vi "Run main.vi"() -> ()   [LabVIEW 2016]
uses:
  Program Files (x86)/National Instruments/LabVIEW 2016/examples/robotics/EPOS2 CANOpen Driver/Low Level VIs/Typedefs/CAN Refnum.ctl
  Program Files (x86)/National Instruments/LabVIEW 2016/examples/robotics/EPOS2 CANOpen Driver/Low Level VIs/Typedefs/CAN Session Pointer.ctl
  Program Files (x86)/National Instruments/LabVIEW 2016/examples/robotics/EPOS2 CANOpen Driver/Low Level VIs/Typedefs/CAN Communication References.ctl
  Program Files (x86)/National Instruments/LabVIEW 2016/examples/robotics/EPOS2 CANOpen Driver/Low Level VIs/Typedefs/kill process notifier array.ctl
  Program Files (x86)/National Instruments/LabVIEW 2016/examples/robotics/EPOS2 CANOpen Driver/Low Level VIs/Typedefs/Write Queue.ctl
  Program Files (x86)/National Instruments/LabVIEW 2016/examples/robotics/EPOS2 CANOpen Driver/Low Level VIs/Typedefs/FPGA CAN Frame Cluster.ctl
  RT/BMS Voltage status 2.ctl
  Tests/BMS Status.ctl
  RT/Pedals Status.ctl
  RT/Clustered SDO.ctl
  RT/Statusword.ctl
  Tests/Dashboard Control.ctl
  RT/Battery Status.ctl
  Tests/Log File Cluster.ctl
  <vilib>/Platform/TimedLoop/XDataNode/timing_clust.ctl
  <vilib>/Platform/TimedLoop/XDataNode/nitl_modes.ctl
  <vilib>/Platform/TimedLoop/XDataNode/wakeup.ctl
  <vilib>/Platform/TimedLoop/XDataNode/XDataNode.xnode
  <vilib>/Platform/TimedLoop/XDataNode/XDNodeRunTimeDep.lvlib
  <vilib>/NI_Real-Time Target Support.lvlib
  <vilib>/RTwatchdog.llb/Watchdog expiration actions.ctl
panel:
  out "Error Notifier":refnum<notifier>
  out "LED Period":i64
  out "LED Color":i16
  out "Last Pedals Update":u32
  in  "Tab Control":T1(tab)
  in  "Don't irritate me":bool=TRUE
  in  "Simulate BMS LV":bool=TRUE
  in  "Simulate Dashboard":bool=TRUE
  in  "Simulate Pedals":bool=TRUE
  in  "Simulate Motors":bool=TRUE
  in  "Simulation Interval":u32=20
  in  "Simulate BMS":bool=TRUE
  in  "\"Pedals\" Status":T2 {"Acceleration pedal" scale=0.0..100.0 scale format="%#_6f%%"; "Break pedal" scale=0.0..100.0 scale format="%#_6f%%"}
  out "Left Motor Status":T3
  out "Target Torque Left":i16(knob) scale=-1000.0..1000.0
  out "Left Motor Statusword":T4
  out "Right Motor Status":T3
  out "Right Motor Statusword":T4
  out "Target Torque Right":i16(knob) scale=1000.0..-1000.0
  out "BMS Status":T5
  out "Battery Status":T6
  out "BMS Low Voltage Status":T7 {"Temp. 0" scale=0.0..80.0; "Temp. 1" scale=0.0..80.0}
  in  "Ready to drive":bool
  in  "Simulate Pumps":bool
  in  "Pumps power":dbl(slide) scale=0.0..100.0 scale format="%#_g%%"
  in  "Dashboard Control":T8={"Tractive System"=TRUE, "RTD"=TRUE, "AMS error"=TRUE, "IMD error"=TRUE, "Low Voltage"=0.0, "High Voltage"=0.0} {"High Voltage" scale=0.0..10.0; "Low Voltage" scale=0.0..10.0}
  in  "Error Listbox":i32(listbox)
  out "Update motors notifier":i32
  out "Update Motors Notifier":refnum<notifier>
  out "Emergency Turn Off Notifier":refnum<notifier>
  out "Pedals status":i32
  out "Update motors":i32
  out "Pool status":i32
  out "Error Queue":refnum<queue>
  out "Shutdown Notifier":refnum<notifier>
  out "Log File Cluster":T9
  out "CAN Session":T11
  out "CANOpen Session":refnum<k20>
  out "Left motor Clustered SDO":T12
  out "Right motor Clustered SDO":T12
  out "State Ring":u16(ring) items=["Init VI", "Init Event Handlers", "Booting sequence", "Operational", "Emergency shutting down", "Shuting down", "Closing VI"]
  in  "Emergency Shutdown Button":bool
  in  "Shutdown Button":bool
  in  "Stop":bool
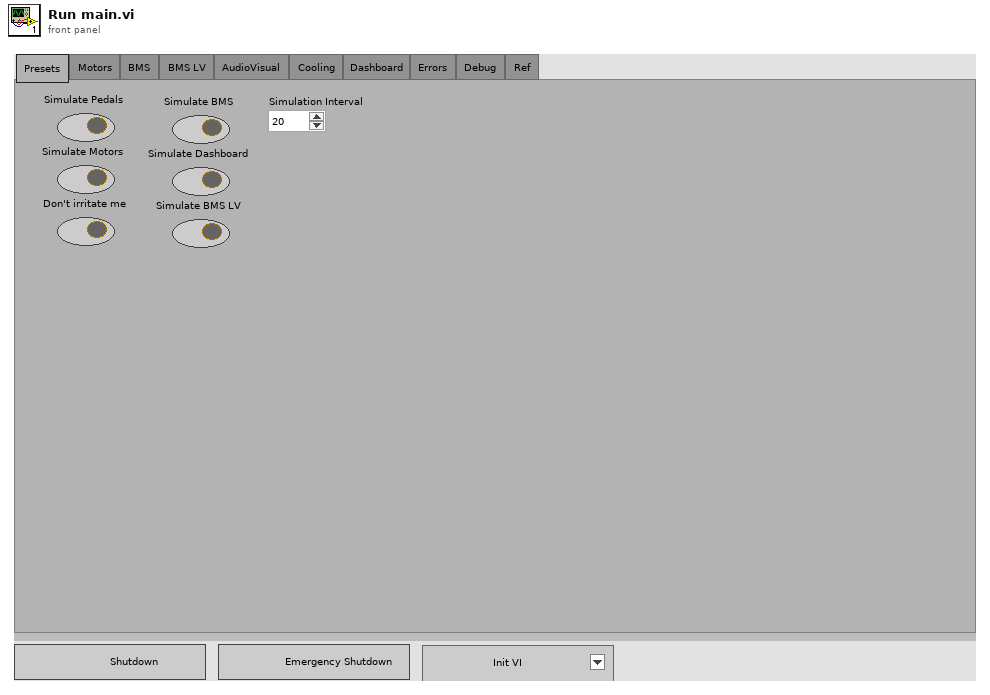
[diagram p1: front panel]
types:
  T1 = enum32{"Presets ", "Motors ", "BMS ", "BMS LV ", "AudioVisual ", "Cooling ", "Dashboard", "Errors ", "Debug ", "Ref "}
  T2 = typedef "Pedals Status.ctl" = cluster{"Acceleration pedal":dbl, "Break pedal":dbl, "Sterring wheel":dbl[unit]}
  T3 = cluster{"Statusword":u16, "Warnings":u16, "Error code":u16, "Error register":u8, "Controller temperature":u8, "Motor temperature":u8, "Troque actual value":i16, "Velocity actual value":i32, "Electric power":u32, "DC current":u32, "Phase A current":u16, "Phase B current":u16, "Electrical Angle":u16}
  T4 = typedef "Statusword.ctl" = cluster{"Ready to switch on":bool, "Switched on":bool, "Operation enabled":bool, "Fault":bool, "Voltage enabled":bool, "Quick stop":bool, "Switch on disabled":bool, "Warning":bool, "Remote":bool, "Target reached":bool, "Internal limit active":bool, "Operation mode specific":bool, "Manufacturer specific":bool}
  T5 = typedef "BMS Status.ctl" = cluster{"INIT":bool, "READY":bool, "WAIT_FOR_ACTIVE":bool, "ACTIVE":bool, "ERROR":bool}
  T6 = typedef "Battery Status.ctl" = cluster{"Hall sensor":i32, "Percent of charge":i16}
  T7 = typedef "BMS Voltage status 2.ctl" = cluster{"Cells Voltage":dbl[], "Temp. 1":u8, "Temp. 0":u8}
  T8 = typedef "Dashboard Control.ctl" = cluster{"Tractive System":bool, "RTD":bool, "AMS error":bool, "IMD error":bool, "Low Voltage":dbl, "High Voltage":dbl}
  T9 = typedef "Log File Cluster.ctl" = cluster{"Log file":refnum<k34>, "semaphore":T10}
  T10 = typedef "Semaphore RefNum" = refnum<k1>
  T11 = typedef "CAN Refnum.ctl" = refnum<k1>
  T12 = typedef "Clustered SDO.ctl" = cluster{"SDO object out":refnum<k20>, "semaphore":T10}
  T13 = typedef "Watchdog expiration actions.ctl" = cluster{"reset":bool, "occurrence":bool, "trigger protocol":enum16{"active high", "active low", "open collector"}, "trigger line":enum16{"none", "line 0", "line 1", "line 2", "line 3", "line 4", "line 5", "line 6", "line 7", "SMB line 0"}, "disable watchdog on VI exit":bool}
  T14 = typedef "XDNodeRunTimeDep.lvlib/timing_clust.ctl" = cluster{"Expected End [f-1]":u64, "Actual End [f-1]":u64, "Finished Late? [f-1]":bool, "Expected End [i-1]":u64, "Actual End [i-1]":u64, "Finished Late? [i-1]":bool, "Expected Start [i]":u64, "Actual Start [i]":u64, "Expected Start [f]":u64, "Actual Start [f]":u64, "Source Name":string, "Structure Name":string, "Period":i64, "Deadline":i64, "Offset":i64, "Start":i64, "Priority":i32, "Timeout":i32, "Mode":T15, "Wakeup Reason":T16, "Error":errorcluster, "Source Type":string, "Secondary Source Type":string, "Global End Time":u64, "Global Start Time":u64, "Frame Duration":u64, "Iteration Duration":u64, "Assigned CPU":i32, "I/O Scan Engine Mode":u32}
  T15 = typedef "XDNodeRunTimeDep.lvlib/nitl_modes.ctl" = enum32{"No Change", "Process missed periods, maintain original phase", "Discard missed periods, maintain original phase", "Process missed periods, ignore original phase", "Discard missed periods, ignore original phase"}
  T16 = typedef "XDNodeRunTimeDep.lvlib/wakeup.ctl" = enum32{"Normal", "Aborted", "Asynchronous wakeup", "Timing source error", "Timed loop error", "Timeout"}
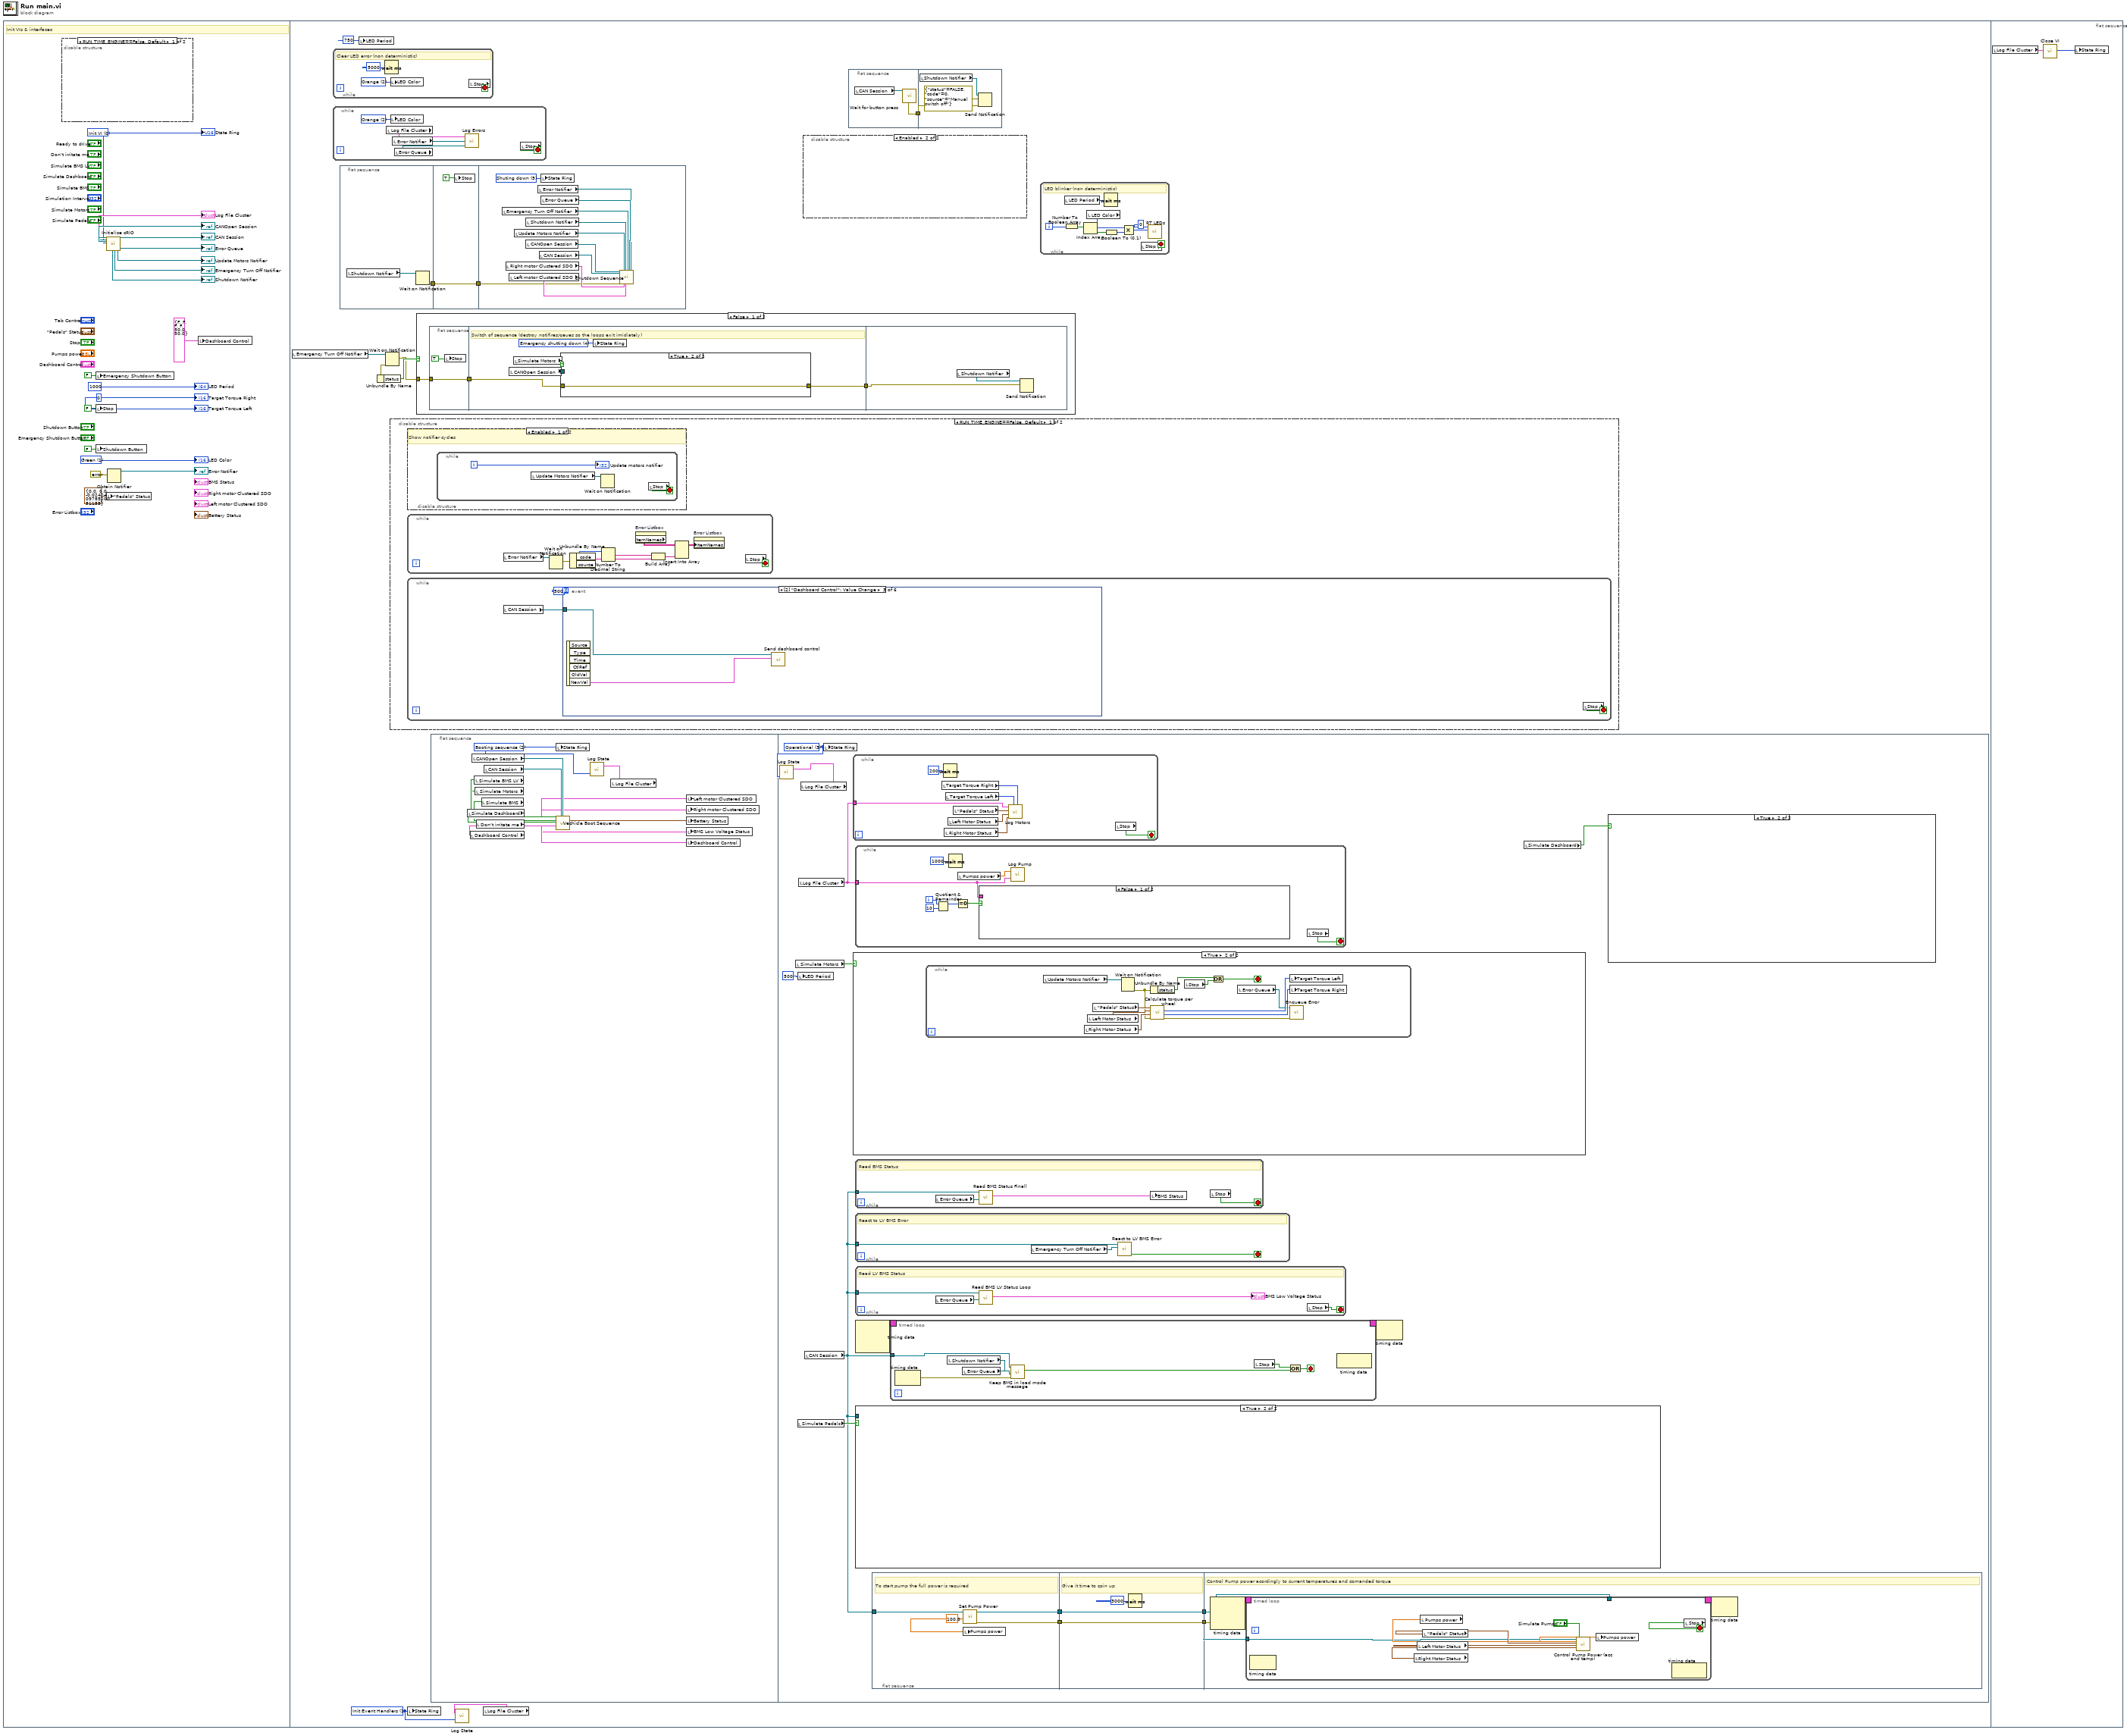
[diagram p0: block diagram]
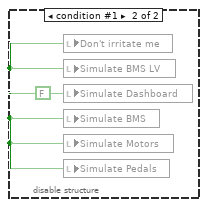
[diagram p2: hidden frame]
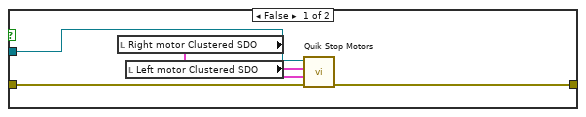
[diagram p3: hidden frame]
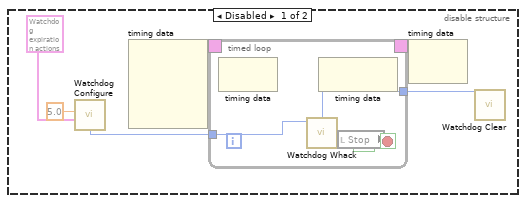
[diagram p5: hidden frame]
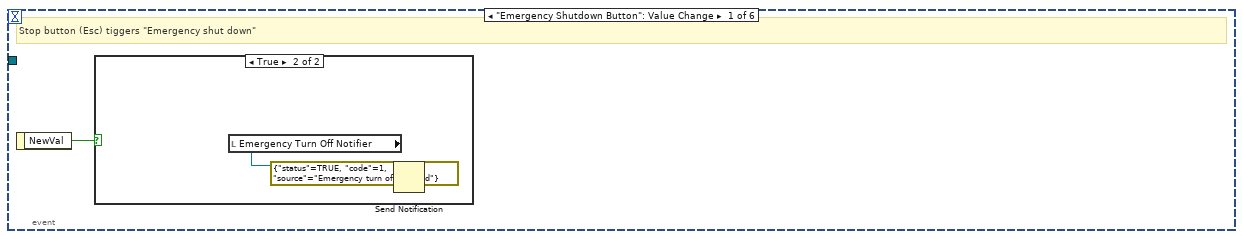
[diagram p7: hidden frame]
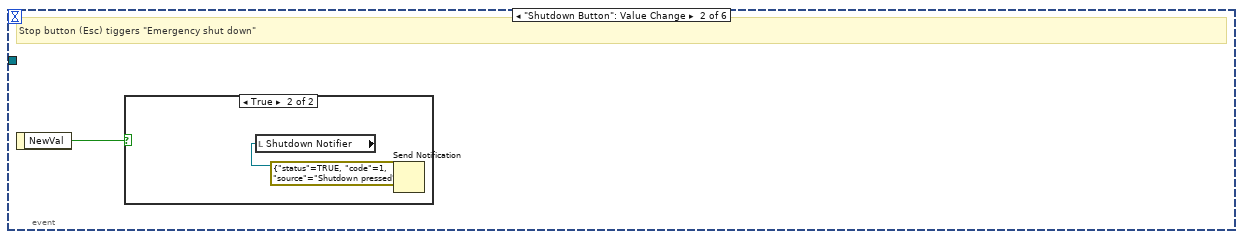
[diagram p9: hidden frame]
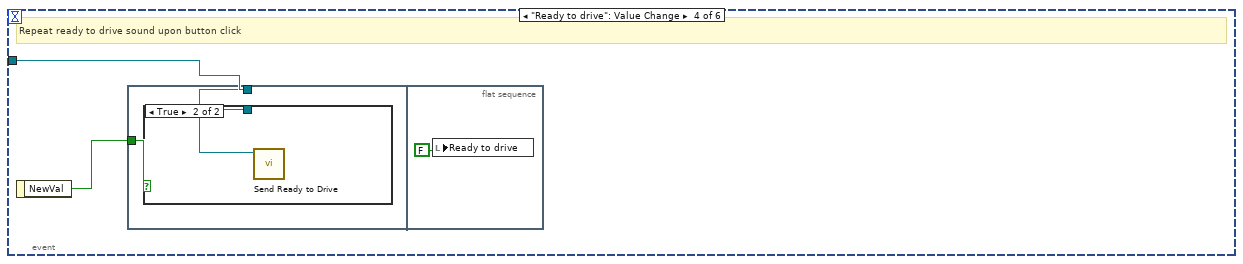
[diagram p11: hidden frame]
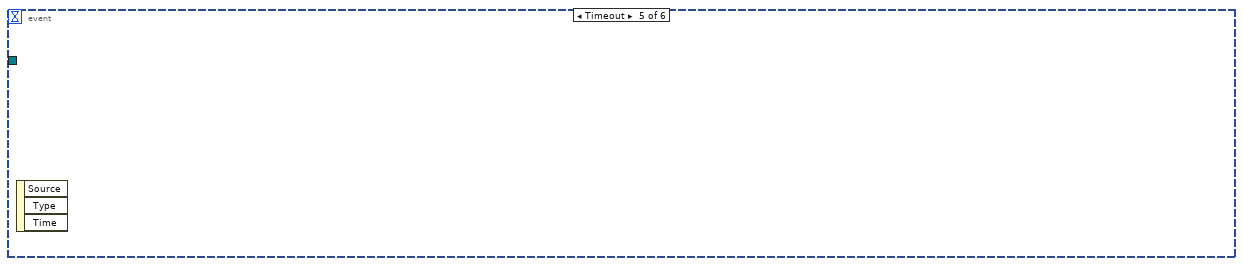
[diagram p13: hidden frame]
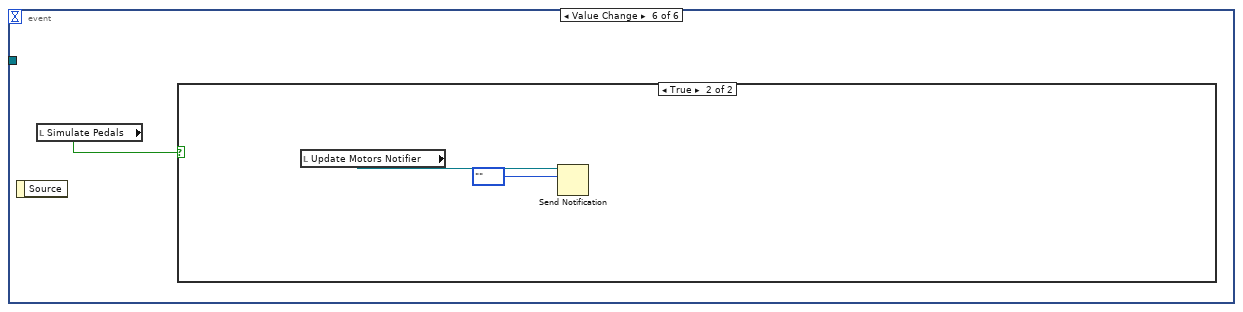
[diagram p14: hidden frame]
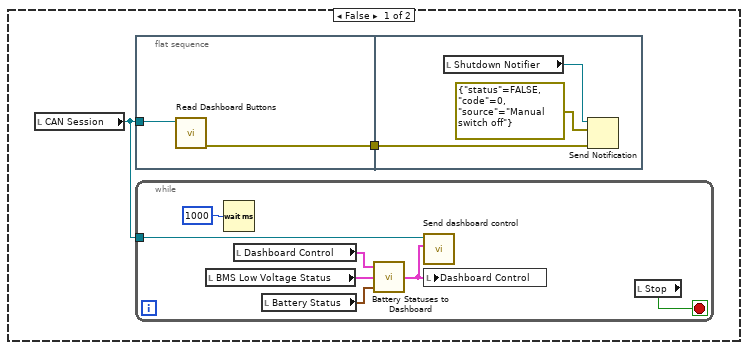
[diagram p17: hidden frame]
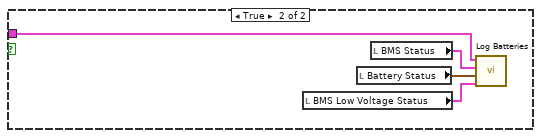
[diagram p18: hidden frame]
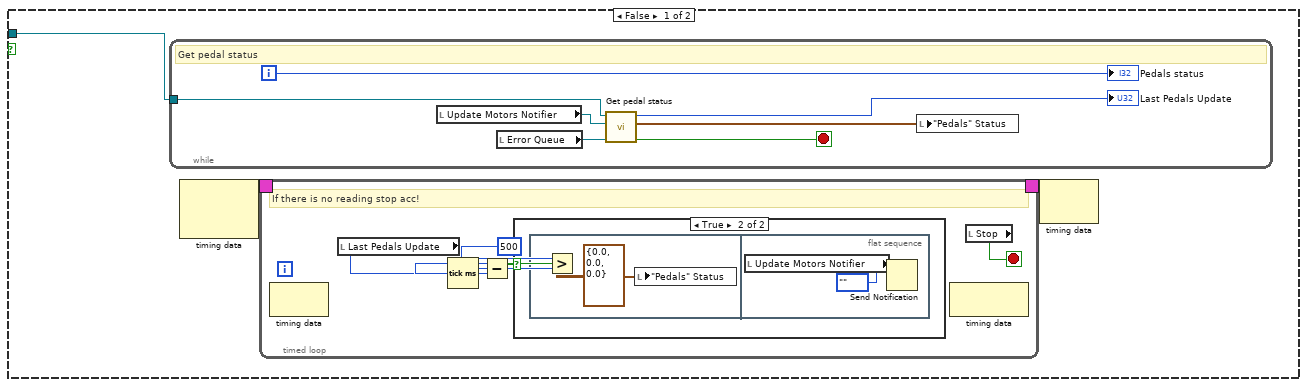
[diagram p19: hidden frame]
diagram:
  n1 = flat-sequence {
    frame #0 {
      w2 = u16 0 items=["Init VI", "Init Event Handlers", "Booting sequence", "Operational", "Emergency shutting down", "Shuting down", "Closing VI"] ("State Ring")
      w10 = u16 1 items=["Green"=1, "Orange"=2]
      w12 = i16 0 ("Target Torque")
      # "Init VIs & interfaces"
      n2 = disable-structure shown="RUN_TIME_ENGINE==False, Default" {
        frame condition #0 (active) {
        }
        frame condition #1 {
          w19 = FALSE ("Don't irritate me")
          n3 = local write "Don't irritate me"(w19) -> ()
          n4 = local write "Simulate BMS LV"(w19) -> ()
          n5 = local write "Simulate Dashboard"(w19) -> ()
          n6 = local write "Simulate BMS"(w19) -> ()
          n7 = local write "Simulate Motors"(w19) -> ()
          n8 = local write "Simulate Pedals"(w19) -> ()
        }
      }
      n9 = local write "Emergency Shutdown Button"(FALSE ("Emergency Shutdown Button")) -> ()
      n10 = local write "Stop"(FALSE ("Stop")) -> ()
      n11 = local write "Shutdown Button"(FALSE ("Shutdown Button")) -> ()
      n12 = call "Initialise cRIO.vi"("State Ring"=w2) -> ("Shutdown Notifier"=→"Shutdown Notifier":refnum<notifier>, "Emergency Turn Off Notifier"=→"Emergency Turn Off Notifier":refnum<notifier>, "Update Motors Notifier"=→"Update Motors Notifier":refnum<notifier>, "Log File Cluster"=→"Log File Cluster":T9, "CANOpen Session"=→"CANOpen Session":refnum<k20>, "CAN Session"=→"CAN Session":T11, "Error Queue"=→"Error Queue":refnum<queue>)  [unwired: 19 in, 1 out]
      n13 = local write "\"Pedals\" Status"(T2 {"Acceleration pedal"=0.0, "Break pedal"=0.0, "Sterring wheel"=-0.024240978520051155} ("\"Pedals\" Status")) -> ()
      n14 = Obtain Notifier(notification data type=errorcluster {"status"=FALSE, "code"=0, "source"=""} ("error constant")) -> (notifier out=→"Error Notifier":refnum<notifier>)  [unwired: 3 in, 2 out]
      n15 = local write "Dashboard Control"(T8 {"Tractive System"=FALSE, "RTD"=FALSE, "AMS error"=FALSE, "IMD error"=FALSE, "Low Voltage"=50.0, "High Voltage"=50.0} ("Dashboard Control")) -> ()
      "Target Torque Left" <- w12
      "Target Torque Right" <- w12
      "LED Color" <- w10
      "LED Period" <- i64 1000 ("LED Period")
      "State Ring" <- w2
    }
    frame #1 {
      w27 = u16 1 items=["Init VI", "Init Event Handlers", "Booting sequence", "Operational", "Emergency shutting down", "Shuting down", "Closing VI"] ("State Ring")
      n16 = local read "Emergency Turn Off Notifier"() -> (w23:refnum<notifier>)
      n17 = while {
        stop <- w76 stop-if-true
        w77 = u16 2 items=["Green"=1, "Orange"=2]
        # "Clear LED error (non deterministic)"
        n18 = Wait (ms)(milliseconds to wait=u32 5000) -> ()  [unwired: 1 out]
        n19 = local write "LED Color"(w77) -> ()
        n20 = local read "Stop"() -> (w76:bool)
      }
      n21 = while {
        stop <- w82 stop-if-true
        w80 = u16 2 items=["Green"=1, "Orange"=2]
        n22 = local read "Log File Cluster"() -> (w79:T9)
        n23 = local write "LED Color"(w80) -> ()
        n24 = local read "Error Notifier"() -> (w78:refnum<notifier>)
        n25 = local read "Error Queue"() -> (w81:refnum<queue>)
        n26 = call "Log Errors.vi"("Error Queue"=w81, "Error Notifier"=w78, "Log File Cluster"=w79) -> ()  [unwired: 1 in]
        n27 = local read "Stop"() -> (w82:bool)
      }
      n28 = flat-sequence {
        tunnel: [w115] -> w25
        tunnel: w25 -> [w118]
        tunnel: [w118] -> w24
        tunnel: w24 -> [w123]
        frame #0 {
          n29 = local read "Shutdown Notifier"() -> (w116:refnum<notifier>)
          n30 = Wait on Notification(notifier=w116) -> (error out=w115:errorcluster)  [unwired: 3 in, 3 out]
        }
        frame #1 {
          n31 = local write "Stop"(TRUE ("Stop")) -> ()
        }
        frame #2 {
          w120 = u16 5 items=["Init VI", "Init Event Handlers", "Booting sequence", "Operational", "Emergency shutting down", "Shuting down", "Closing VI"] ("State Ring")
          n32 = local read "Emergency Turn Off Notifier"() -> (w121:refnum<notifier>)
          n33 = local read "Right motor Clustered SDO"() -> (w124:T12)
          n34 = local read "Left motor Clustered SDO"() -> (w125:T12)
          n35 = local read "Update Motors Notifier"() -> (w127:refnum<notifier>)
          n36 = local read "Shutdown Notifier"() -> (w126:refnum<notifier>)
          n37 = local read "CANOpen Session"() -> (w129:refnum<k20>)
          n38 = local read "Error Notifier"() -> (w119:refnum<notifier>)
          n39 = local read "CAN Session"() -> (w128:T11)
          n40 = local write "State Ring"(w120) -> ()
          n41 = local read "Error Queue"() -> (w122:refnum<queue>)
          n42 = call "Shutdown Sequence.vi"("CANOpen Session"=w129, "CAN Session"=w128, "error in (no error)"=w123, "Update Motors Notifier"=w127, "Right motor Clustered SDO"=w124, "Shutdown Notifier"=w126, "Left motor Clustered SDO"=w125, "Emergency Turn Off Notifier"=w121, "Error Queue"=w122, "Error Notifier"=w119) -> ()  [unwired: 17 in, 1 out]
        }
      }
      n43 = local write "LED Period"(i64 750 ("LED Period")) -> ()
      n44 = Wait on Notification(notifier=w23) -> (notification=w20:errorcluster, error out=w22:errorcluster)  [unwired: 3 in, 2 out]
      n45 = Unbundle By Name(w22) -> ("status"=w21:bool)
      n46 = disable-structure shown="RUN_TIME_ENGINE==False, Default" {
        frame condition #0 (active) {
          n47 = disable-structure shown="Enabled" {
            frame Enabled {
              # "Show notifier cycles"
              n48 = while {
                i -> [w92]
                stop <- w93 stop-if-true
                n49 = local read "Update Motors Notifier"() -> (w94:refnum<notifier>)
                n50 = Wait on Notification(notifier=w94) -> ()  [unwired: 3 in, 4 out]
                n51 = local read "Stop"() -> (w93:bool)
                "Update motors notifier" <- w92
              }
            }
            frame Disabled {
            }
          }
          n52 = while {
            stop <- w83 stop-if-true
            n53 = local read "Error Notifier"() -> (w91:refnum<notifier>)
            n54 = Wait on Notification(notifier=w91) -> (notification=w90:errorcluster)  [unwired: 3 in, 3 out]
            n55 = Unbundle By Name(w90) -> ("code"=w87:i32, "source"=w89:string)
            n56 = Number To Decimal String(number=w87) -> (decimal integer string=w88:string)  [unwired: 1 in]
            n57 = property on="Error Listbox" class="MCListbox (strict)"() -> ("ItemNames"=w85:string[][])  [unwired: 2 in, 2 out]
            n58 = Build Array(w88, w89) -> (w86:string[])
            n59 = Insert Into Array(array=w85, new element=w86) -> (w84:string[][])  [unwired: 2 in]
            n60 = property on="Error Listbox" class="MCListbox (strict)"("ItemNames"=w84) -> ()  [unwired: 2 in, 2 out]
            n61 = local read "Stop"() -> (w83:bool)
          }
          n62 = while {
            stop <- w96 stop-if-true
            n63 = local read "CAN Session"() -> (w97:T11)
            n64 = event shown="[2] \"Dashboard Control\": Value Change" {
              selector: _ -> [_ _ _ _ _ _]
              dyn-events: _ -> [_ _ _ _ _ _]
              timeout: 500 -> [_ _ _ _ _ _]
              tunnel: w97 -> [_ _ w104 w106 _ _]
              event "Emergency Shutdown Button": Value Change {
                # "Stop button (Esc) tiggers \"Emergency shut down\""
                n65 = event-data() -> ("NewVal"=w98:bool)  [unwired: 1 in]
                n66 = case shown="True" w98 {
                  frame False {
                  }
                  frame True {
                    n67 = local read "Emergency Turn Off Notifier"() -> (w100:refnum<notifier>)
                    n68 = Send Notification(notification=errorcluster {"status"=TRUE, "code"=1, "source"="Emergency turn off pressed"}, notifier=w100) -> ()  [unwired: 1 in, 2 out]
                  }
                }
              }
              event "Shutdown Button": Value Change {
                # "Stop button (Esc) tiggers \"Emergency shut down\""
                n69 = event-data() -> ("NewVal"=w101:bool)  [unwired: 1 in]
                n70 = case shown="True" w101 {
                  frame False {
                  }
                  frame True {
                    n71 = local read "Shutdown Notifier"() -> (w103:refnum<notifier>)
                    n72 = Send Notification(notification=errorcluster {"status"=TRUE, "code"=1, "source"="Shutdown pressed"}, notifier=w103) -> ()  [unwired: 1 in, 2 out]
                  }
                }
              }
              event Value Change {
                n73 = event-data() -> ("NewVal"=w105:T8)  [unwired: 1 in, 5 out]
                n74 = call "Send dashboard control.vi"("Dashboard Control"=w105, "CAN Session In"=w104) -> ()  [unwired: 8 in, 2 out]
              }
              event "Ready to drive": Value Change {
                # "Repeat ready to drive sound upon button click"
                n75 = event-data() -> ("NewVal"=w107:bool)  [unwired: 1 in]
                n76 = flat-sequence {
                  tunnel: w107 -> [w109]
                  tunnel: w106 -> [w108]
                  frame #0 {
                    n77 = case shown="True" w109 {
                      tunnel: w108 -> [_ w110]
                      frame False {
                      }
                      frame True {
                        n78 = call "Send Ready to Drive.vi"("CAN Session In"=w110) -> ()  [unwired: 9 in, 2 out]
                      }
                    }
                  }
                  frame #1 {
                    n79 = local write "Ready to drive"(FALSE ("Ready to drive")) -> ()
                  }
                }
              }
              event Timeout {
                n80 = event-data() -> ()  [unwired: 1 in, 3 out]
              }
              event Value Change {
                n81 = event-data() -> ()  [unwired: 1 in, 1 out]
                n82 = local read "Simulate Pedals"() -> (w112:bool)
                n83 = case shown="True" w112 {
                  frame False {
                  }
                  frame True {
                    n84 = local read "Update Motors Notifier"() -> (w113:refnum<notifier>)
                    n85 = Send Notification(notification=enum16{""}."", notifier=w113) -> ()  [unwired: 1 in, 2 out]
                  }
                }
              }
            }
            n86 = local read "Stop"() -> (w96:bool)
          }
        }
        frame condition #1 {
        }
      }
      n87 = local write "State Ring"(w27) -> ()
      n88 = case shown="False" w21 {
        tunnel: w20 -> [w30 _]
        frame False {
          n89 = flat-sequence {
            tunnel: [w33] -> w32
            tunnel: w30 -> [w33]
            tunnel: w32 -> [w35]
            tunnel: [w37] -> w31
            tunnel: w31 -> [w46]
            frame #0 {
              n90 = local write "Stop"(TRUE ("Stop")) -> ()
            }
            frame #1 {
              w36 = u16 4 items=["Init VI", "Init Event Handlers", "Booting sequence", "Operational", "Emergency shutting down", "Shuting down", "Closing VI"] ("State Ring")
              # "Switch of sequence (destroy notifires/qeues so the loops exit imidiately)"
              n91 = local read "CANOpen Session"() -> (w38:refnum<k20>)
              n92 = local read "Simulate Motors"() -> (w39:bool)
              n93 = case shown="True" w39 {
                tunnel: w38 -> [w44 _]
                tunnel: [w41 w45] -> w37
                tunnel: w35 -> [w40 w45]
                frame False {
                  n94 = local read "Right motor Clustered SDO"() -> (w42:T12)
                  n95 = local read "Left motor Clustered SDO"() -> (w43:T12)
                  n96 = call "Quik Stop Motors.vi"("error in (no error)"=w40, "Left motor Clustered SDO"=w43, "Right motor Clustered SDO"=w42, "CANOpen session"=w44) -> ("error out"=w41:errorcluster)  [unwired: 5 in, 2 out]
                }
                frame True {
                }
              }
              n97 = local write "State Ring"(w36) -> ()
            }
            frame #2 {
              n98 = local read "Shutdown Notifier"() -> (w47:refnum<notifier>)
              n99 = Send Notification(notification=w46, notifier=w47) -> ()  [unwired: 1 in, 2 out]
            }
          }
        }
        frame True {
        }
      }
      n100 = flat-sequence {
        frame #0 {
          w131 = u16 2 items=["Init VI", "Init Event Handlers", "Booting sequence", "Operational", "Emergency shutting down", "Shuting down", "Closing VI"] ("State Ring")
          n101 = local read "Simulate Dashboard"() -> (w141:bool)
          n102 = local read "Dashboard Control"() -> (w133:T8)
          n103 = local read "CANOpen Session"() -> (w138:refnum<k20>)
          n104 = local read "Simulate BMS LV"() -> (w144:bool)
          n105 = local read "Simulate Motors"() -> (w142:bool)
          n106 = local read "Don't irritate me"() -> (w140:bool)
          n107 = local read "Simulate BMS"() -> (w143:bool)
          n108 = local read "CAN Session"() -> (w139:T11)
          n109 = local write "State Ring"(w131) -> ()
          n110 = call "Vechicle Boot Sequence.vi"("Simulate BMS LV"=w144, "Simulate Motors"=w142, "Simulate BMS"=w143, "Simulate Dashboard"=w141, "Don't irritate me"=w140, "Dashboard Control in"=w133, "CAN Session"=w139, "CANOpen Session"=w138) -> ("Left motor Clustered SDO"=w136:T12, "Right motor Clustered SDO"=w137:T12, "Battery Status"=w135:T6, "BMS Low Voltage Status"=w132:T7, "Dashboard Control out"=w134:T8)  [unwired: 14 in, 1 out]
          n111 = local read "Log File Cluster"() -> (w130:T9)
          n112 = call "Log State.vi"("State Ring"=w131, "Log File Cluster"=w130) -> ()  [unwired: 1 in]
          n113 = local write "Left motor Clustered SDO"(w136) -> ()
          n114 = local write "Right motor Clustered SDO"(w137) -> ()
          n115 = local write "Battery Status"(w135) -> ()
          n116 = local write "BMS Low Voltage Status"(w132) -> ()
          n117 = local write "Dashboard Control"(w134) -> ()
        }
        frame #1 {
          w146 = u16 3 items=["Init VI", "Init Event Handlers", "Booting sequence", "Operational", "Emergency shutting down", "Shuting down", "Closing VI"] ("State Ring")
          n118 = local read "Simulate Motors"() -> (w152:bool)
          n119 = local read "Simulate Pedals"() -> (w151:bool)
          n120 = local write "LED Period"(i64 500 ("LED Period")) -> ()
          n121 = local read "Log File Cluster"() -> (w148:T9)
          n122 = local read "Log File Cluster"() -> (w147:T9)
          n123 = call "Log State.vi"("State Ring"=w146, "Log File Cluster"=w147) -> ()  [unwired: 1 in]
          n124 = local read "CAN Session"() -> (w150:T11)
          n125 = local write "State Ring"(w146) -> ()
          n126 = while {
            tunnel: w148 -> [w185]
            stop <- w186 stop-if-true
            n127 = local read "Target Torque Right"() -> (w188:i16)
            n128 = Wait (ms)(milliseconds to wait=u32 200) -> ()  [unwired: 1 out]
            n129 = local read "Right Motor Status"() -> (w190:T3)
            n130 = local read "Target Torque Left"() -> (w189:i16)
            n131 = local read "Left Motor Status"() -> (w191:T3)
            n132 = local read "\"Pedals\" Status"() -> (w192:T2)
            n133 = call "Log Motors.vi"("Target Torque Right"=w188, "Target Torque Left"=w189, "Right Motor Status"=w190, "Left Motor Status"=w191, "\"Pedals\" Status"=w192, "Log File Cluster"=w185) -> ()  [unwired: 4 in]
            n134 = local read "Stop"() -> (w186:bool)
          }
          n135 = case shown="True" w152 {
            frame False {
              n136 = local read "Right motor Clustered SDO"() -> (w266:T12)
              n137 = local read "Left motor Clustered SDO"() -> (w267:T12)
              n138 = while {
                tunnel: w267 -> [w287]
                tunnel: w266 -> [w288]
                i -> [w290]
                stop <- w281 stop-if-true
                # "Update motors target values"
                n139 = local read "Update Motors Notifier"() -> (w289:refnum<notifier>)
                n140 = local read "Right Motor Status"() -> (w284:T3)
                n141 = local read "Left Motor Status"() -> (w285:T3)
                n142 = local read "\"Pedals\" Status"() -> (w286:T2)
                n143 = call "Update motors target values.vi"("Update Motors Notifier"=w289, "Right motor Clustered SDO"=w288, "Left motor Clustered SDO"=w287, "\"Pedals\" Status"=w286, "Left Motor Status"=w285, "Right Motor Status"=w284) -> ("Target Torque Left"=w283:i16, "Target Torque Right"=w282:i16, "Exit?"=w281:bool)  [unwired: 19 in]
                n144 = local write "Target Torque Left"(w283) -> ()
                n145 = local write "Target Torque Right"(w282) -> ()
                "Update motors" <- w290
              }
              n146 = node-c288() -> (w265:T14)  [unwired: 3 in]
              n147 = timed-loop {
                timing: w265 -> [_]
                timing-out: [_] -> w264
                tunnel: w267 -> [w275]
                tunnel: w266 -> [w274]
                i -> [w276]
                stop <- w268 stop-if-true
                # "Pool motor status"
                n148 = node-c288() -> ()  [unwired: 1 in, 2 out]
                n149 = local read "Update Motors Notifier"() -> (w273:refnum<notifier>)
                n150 = call "Pool motor status.vi"("Update Motors Notifier"=w273, "Right motor Clustered SDO"=w274, "Left motor Clustered SDO"=w275) -> ("Left Motor Status"=→"Left Motor Status":T3, "Left Motor Statusword"=→"Left Motor Statusword":T4, "Right Motor Status"=→"Right Motor Status":T3, "Right Motor Statusword"=→"Right Motor Statusword":T4, "Exit?"=w268:bool)  [unwired: 20 in]
                n151 = node-c288() -> ()  [unwired: 1 in, 1 out]
                "Pool status" <- w276
              }
              n152 = node-c288(w264) -> ()  [unwired: 1 out]
            }
            frame True {
              n153 = while {
                stop <- w298 stop-if-true
                n154 = local read "Update Motors Notifier"() -> (w300:refnum<notifier>)
                n155 = local read "Right Motor Status"() -> (w295:T3)
                n156 = local read "Left Motor Status"() -> (w296:T3)
                n157 = local read "\"Pedals\" Status"() -> (w297:T2)
                n158 = Wait on Notification(notifier=w300) -> (error out=w291:errorcluster)  [unwired: 3 in, 3 out]
                n159 = Unbundle By Name(w291) -> ("status"=w292:bool)
                n160 = call "Calculate torque per wheel.vi"("Error In"=w291, "Right Motor Status"=w295, "Left Motor Status"=w296, "\"Pedals\" Status"=w297) -> ("Error Out"=w294:errorcluster, "Target Torque Right"=w301:i16, "Target Torque Left"=w302:i16)  [unwired: 5 in]
                n161 = local read "Stop"() -> (w299:bool)
                n162 = Or(x=w292, y=w299) -> (x .or. y?=w298:bool)
                n163 = local read "Error Queue"() -> (w293:refnum<queue>)
                n164 = local write "Target Torque Left"(w302) -> ()
                n165 = local write "Target Torque Right"(w301) -> ()
                n166 = call "Enqueue Error.vi"("error in"=w294, "Error Queue"=w293) -> ()  [unwired: 10 in]
              }
            }
          }
          n167 = while {
            tunnel: w148 -> [w173]
            i -> [w179]
            stop <- w180 stop-if-true
            n168 = Quotient & Remainder(x=w179, y=10) -> (x-y*floor(x/y)=w176:i32)  [unwired: 1 out]
            n169 = Wait (ms)(milliseconds to wait=u32 1000) -> ()  [unwired: 1 out]
            n170 = Equal To 0?(x=w176) -> (x = 0?=w175:bool)
            n171 = local read "Pumps power"() -> (w174:dbl)
            n172 = case shown="False" w175 {
              tunnel: w173 -> [_ w181]
              frame False {
              }
              frame True {
                n173 = local read "BMS Low Voltage Status"() -> (w183:T7)
                n174 = local read "Battery Status"() -> (w182:T6)
                n175 = local read "BMS Status"() -> (w184:T5)
                n176 = call "Log Batteries.vi"("BMS Low Voltage Status"=w183, "Battery Status"=w182, "BMS Status"=w184, "Log File Cluster"=w181) -> ()  [unwired: 6 in]
              }
            }
            n177 = call "Log Pump.vi"("Log File Cluster"=w173, "Pumps power"=w174) -> ()  [unwired: 1 in]
            n178 = local read "Stop"() -> (w180:bool)
          }
          n179 = while {
            tunnel: w150 -> [w195]
            stop <- w194 stop-if-true
            # "Read BMS Status"
            n180 = local read "Error Queue"() -> (w193:refnum<queue>)
            n181 = call "Read BMS Status Finall.vi"("Error Queue"=w193, "CAN Session In"=w195) -> ("BMS Status"=w196:T5)  [unwired: 8 in, 1 out]
            n182 = local write "BMS Status"(w196) -> ()
            n183 = local read "Stop"() -> (w194:bool)
          }
          n184 = while {
            tunnel: w150 -> [w249]
            stop <- w251 stop-if-true
            # "React to LV BMS Error"
            n185 = local read "Emergency Turn Off Notifier"() -> (w250:refnum<notifier>)
            n186 = call "React to LV BMS Error.vi"("Emergency Turn Off Notifier"=w250, "CAN Session In"=w249) -> ("Exit?"=w251:bool)  [unwired: 8 in, 1 out]
          }
          n187 = while {
            tunnel: w150 -> [w199]
            stop <- w197 stop-if-true
            # "Read LV BMS Status"
            n188 = local read "Error Queue"() -> (w198:refnum<queue>)
            n189 = call "Read BMS LV Status Loop.vi"("Error Queue"=w198, "CAN Session In"=w199) -> ("BMS Low Voltage Status"=→"BMS Low Voltage Status":T7)  [unwired: 8 in, 1 out]
            n190 = local read "Stop"() -> (w197:bool)
          }
          n191 = node-c288() -> (w158:T14)  [unwired: 3 in]
          n192 = case shown="True" w151 {
            tunnel: w150 -> [w226 _]
            frame False {
              n193 = while {
                tunnel: w226 -> [w242]
                i -> [w248]
                stop <- w243 stop-if-true
                # "Get pedal status"
                n194 = local read "Update Motors Notifier"() -> (w245:refnum<notifier>)
                n195 = local read "Error Queue"() -> (w246:refnum<queue>)
                n196 = call "Get pedal status.vi"("Error Queue"=w246, "Update Motors Notifier"=w245, "CAN Session In"=w242) -> ("Exit?"=w243:bool, "\"Pedals\" Status"=w244:T2, "Last Pedals Update"=→"Last Pedals Update":u32)  [unwired: 6 in]
                n197 = local write "\"Pedals\" Status"(w244) -> ()
                "Pedals status" <- w248
              }
              n198 = node-c288() -> (w228:T14)  [unwired: 2 in]
              n199 = timed-loop {
                timing: w228 -> [_]
                timing-out: [_] -> w227
                stop <- w229 stop-if-true
                # "If there is no reading stop acc!"
                n200 = node-c288() -> ()  [unwired: 1 in, 1 out]
                n201 = local read "Last Pedals Update"() -> (w233:u32)
                n202 = Tick Count (ms)() -> (millisecond timer value=w234:u32)
                n203 = Subtract(x=w234, y=w233) -> (x-y=w232:u32)
                n204 = Greater?(x=w232, y=u32 500) -> (0:w230:bool)
                n205 = case shown="True" w230 {
                  frame False {
                  }
                  frame True {
                    n206 = flat-sequence {
                      frame #0 {
                        n207 = local write "\"Pedals\" Status"(T2 {"Acceleration pedal"=0.0, "Break pedal"=0.0, "Sterring wheel"=0.0} ("\"Pedals\" Status")) -> ()
                      }
                      frame #1 {
                        n208 = local read "Update Motors Notifier"() -> (w236:refnum<notifier>)
                        n209 = Send Notification(notification=enum16{""}."", notifier=w236) -> ()  [unwired: 1 in, 2 out]
                      }
                    }
                  }
                }
                n210 = node-c288() -> ()  [unwired: 1 in, 1 out]
                n211 = local read "Stop"() -> (w229:bool)
              }
              n212 = node-c288(w227) -> ()  [unwired: 1 out]
            }
            frame True {
            }
          }
          n213 = flat-sequence {
            tunnel: [w204] -> w156
            tunnel: [w203] -> w155
            tunnel: w150 -> [w201]
            tunnel: w156 -> [w206]
            tunnel: [w206] -> w154
            tunnel: [w205] -> w153
            tunnel: w155 -> [w205]
            tunnel: w154 -> [w208]
            tunnel: w153 -> [w209]
            frame #0 {
              w202 = 100.0 ("Power %")
              # "To start pump the full power is required"
              n214 = call "Set Pump Power.vi"("Power %"=w202, "CAN Session In"=w201) -> ("error out"=w203:errorcluster, "CAN Session Out"=w204:T11)  [unwired: 8 in]
              n215 = local write "Pumps power"(w202) -> ()
            }
            frame #1 {
              # "Give it time to spin up"
              n216 = Wait (ms)(milliseconds to wait=u32 3000) -> ()  [unwired: 1 out]
            }
            frame #2 {
              # "Control Pump power acordingly to current temperatures and comanded torque"
              n217 = node-c288(w209) -> (w211:T14)  [unwired: 2 in]
              n218 = timed-loop {
                timing: w211 -> [_]
                timing-out: [_] -> w210
                tunnel: w208 -> [_]
                tunnel: w208 -> [w213]
                stop <- w212 stop-if-true
                n219 = node-c288() -> ()  [unwired: 1 in, 1 out]
                n220 = local read "Right Motor Status"() -> (w217:T3)
                n221 = local read "Left Motor Status"() -> (w218:T3)
                n222 = local read "Pumps power"() -> (w215:dbl)
                n223 = local read "\"Pedals\" Status"() -> (w219:T2)
                n224 = call "Control Pump Power (acc and temp).vi"("CAN Session In"=w213, "Pumps power in"=w215, "\"Pedals\" Status"=w219, "Left Motor Status"=w218, "Right Motor Status"=w217, "Simulate Pumps"="Simulate Pumps") -> ("Pumps power out"=w214:dbl)  [unwired: 11 in, 2 out]
                n225 = local write "Pumps power"(w214) -> ()
                n226 = node-c288() -> ()  [unwired: 1 in, 1 out]
                n227 = local read "Stop"() -> (w212:bool)
              }
              n228 = node-c288(w210) -> ()  [unwired: 1 out]
            }
          }
          n229 = timed-loop {
            timing: w158 -> [_]
            timing-out: [_] -> w157
            tunnel: w150 -> [w257]
            stop <- w252 stop-if-true
            n230 = node-c288() -> (w258:errorcluster)  [unwired: 1 in]
            n231 = local read "Shutdown Notifier"() -> (w253:refnum<notifier>)
            n232 = local read "Error Queue"() -> (w254:refnum<queue>)
            n233 = call "Keep BMS in load mode message.vi"("error in"=w258, "Error Queue"=w254, "Shutdown Notifier"=w253, "CAN Session In"=w257) -> ("Exit?"=w256:bool)  [unwired: 6 in, 1 out]
            n234 = local read "Stop"() -> (w255:bool)
            n235 = Or(x=w255, y=w256) -> (x .or. y?=w252:bool)
            n236 = node-c288() -> ()  [unwired: 1 in, 1 out]
          }
          n237 = node-c288(w157) -> ()  [unwired: 1 out]
          n238 = local read "Simulate Dashboard"() -> (w145:bool)
          n239 = case shown="True" w145 {
            frame False {
              n240 = local read "CAN Session"() -> (w159:T11)
              n241 = flat-sequence {
                tunnel: [w169] -> w160
                tunnel: w159 -> [w168]
                tunnel: w160 -> [w170]
                frame #0 {
                  n242 = call "Read Dashboard Buttons.vi"("CAN Session In"=w168) -> ("error out"=w169:errorcluster)  [unwired: 7 in, 3 out]
                }
                frame #1 {
                  n243 = local read "Shutdown Notifier"() -> (w171:refnum<notifier>)
                  n244 = Send Notification(notification=errorcluster {"status"=FALSE, "code"=0, "source"="Manual switch off"}, notifier=w171, error in (no error)=w170) -> ()  [unwired: 2 out]
                }
              }
              n245 = while {
                tunnel: w159 -> [w163]
                stop <- w162 stop-if-true
                n246 = local read "BMS Low Voltage Status"() -> (w164:T7)
                n247 = Wait (ms)(milliseconds to wait=u32 1000) -> ()  [unwired: 1 out]
                n248 = local read "Dashboard Control"() -> (w166:T8)
                n249 = local read "Battery Status"() -> (w165:T6)
                n250 = call "Battery Statuses to Dashboard.vi"("Battery Status"=w165, "BMS Low Voltage Status"=w164, "Dashboard Control in"=w166) -> ("Dashboard Control out"=w161:T8)
                n251 = call "Send dashboard control.vi"("Dashboard Control"=w161, "CAN Session In"=w163) -> ()  [unwired: 8 in, 2 out]
                n252 = local write "Dashboard Control"(w161) -> ()
                n253 = local read "Stop"() -> (w162:bool)
              }
            }
            frame True {
            }
          }
        }
      }
      n254 = local read "Log File Cluster"() -> (w26:T9)
      n255 = call "Log State.vi"("State Ring"=w27, "Log File Cluster"=w26) -> ()  [unwired: 1 in]
      n256 = disable-structure shown="Enabled" {
        frame Disabled {
          n257 = call <vilib>:"Watchdog Configure.vi"("expiration actions"=T13 {"reset"=TRUE, "occurrence"=FALSE, "trigger protocol"=enum."active high", "trigger line"=enum."none", "disable watchdog on VI exit"=TRUE}, "timeout (1 sec)"=5.0) -> ("watchdogID"=w50:u64)  [unwired: 2 in, 3 out]
          n258 = node-c288() -> (w53:T14)  [unwired: 4 in]
          n259 = timed-loop {
            timing: w53 -> [_]
            timing-out: [_] -> w52
            tunnel: w50 -> [w56]
            tunnel: [w55] -> w51
            stop <- w54 stop-if-true
            n260 = node-c288() -> ()  [unwired: 1 in, 1 out]
            n261 = call <vilib>:"Watchdog Whack.vi"("watchdogID in"=w56) -> ("watchdogID out"=w55:u64)  [unwired: 4 in, 2 out]
            n262 = node-c288() -> ()  [unwired: 1 in, 1 out]
            n263 = local read "Stop"() -> (w54:bool)
          }
          n264 = node-c288(w52) -> ()  [unwired: 1 out]
          n265 = call <vilib>:"Watchdog Clear.vi"("watchdogID in"=w51) -> ()  [unwired: 6 in, 1 out]
        }
        frame Enabled {
        }
      }
      n266 = flat-sequence {
        tunnel: [w70] -> w28
        tunnel: w28 -> [w72]
        frame #0 {
          n267 = local read "CAN Session"() -> (w71:T11)
          n268 = call "Wait for button press.vi"("CAN Session In"=w71) -> ("error out"=w70:errorcluster)  [unwired: 10 in]
        }
        frame #1 {
          n269 = local read "Shutdown Notifier"() -> (w74:refnum<notifier>)
          n270 = Send Notification(notification=errorcluster {"status"=FALSE, "code"=0, "source"="Manual switch off"}, notifier=w74, error in (no error)=w72) -> ()  [unwired: 2 out]
        }
      }
      n271 = while {
        i -> [w67]
        stop <- w69 stop-if-true
        # "LED blinker (non deterministic)"
        n272 = local read "LED Period"() -> (w61:i64)
        n273 = Number To Boolean Array(number=w67) -> (Boolean array=w66:bool[])
        n274 = Index Array(array=w66) -> (element=w65:bool)  [unwired: 1 in]
        n275 = local read "LED Color"() -> (w63:i16)
        n276 = Wait (ms)(milliseconds to wait=w61) -> ()  [unwired: 1 out]
        n277 = Boolean To (0,1)(Boolean=w65) -> (0, 1=w64:i16)
        n278 = Multiply(x=w63, y=w64) -> (x*y=w62:i16)
        n279 = local read "Stop"() -> (w69:bool)
        n280 = call <vilib>:"RT LEDs.vi"("State"=w62, "LED Num"=0) -> ()  [unwired: 4 in, 2 out]
      }
    }
    frame #2 {
      n281 = local read "Log File Cluster"() -> (w303:T9)
      n282 = call "Close VI.vi"("Log File Cluster"=w303) -> ("State Ring"=w304:u16)  [unwired: 10 in]
      n283 = local write "State Ring"(w304) -> ()
    }
  }
